vi "Init_TextMark.vi"() -> (0 "TextMark out":T1)   [LabVIEW 2016]
uses:
  <vilib>/Instr/_visa.llb/VISA Open Access Mode.ctl
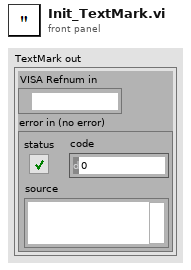
[diagram p1: front panel]
types:
  T1 = cluster{"VISA Refnum in":refnum<visa-resource-name>, "error in (no error)":errorcluster}
  T2 = typedef "VISA Open Access Mode.ctl" = u32
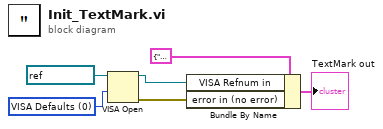
[diagram p0: block diagram]
diagram:
  w2 = T2 0 items=["VISA Defaults"=0, "Exclusive Lock"=1, "Load Configured Settings"=4] ("Access Mode")
  n1 = VISA Open(access mode=w2, VISA resource name=refnum<visa-resource-name> "COM11") -> (VISA resource name=w3:refnum<visa-resource-name>, error out=w4:errorcluster)  [unwired: 3 in]
  n2 = Bundle By Name(cluster=T1 {"VISA Refnum in"="", "error in (no error)"={"status"=FALSE, "code"=0, "source"=""}} ("TextMark out"), "VISA Refnum in"=w3, "error in (no error)"=w4) -> (→"TextMark out":T1)
